vi "SmartSyntax to FormatString.vi"(0 "functionbase in":refnum<class "functionbase.lvclass">, 5 "String":string, 11 "error in (no error)":errorcluster) -> (4 "functionbase out":refnum<class "functionbase.lvclass">, 6 "Scan Syntax Format":T1, 15 "error out":errorcluster)   [LabVIEW 2019, in "LSL.lvlib" / "functionbase.lvclass"]
uses:
  functionbase.lvclass
  common/function utils/Scan Syntax Format.ctl
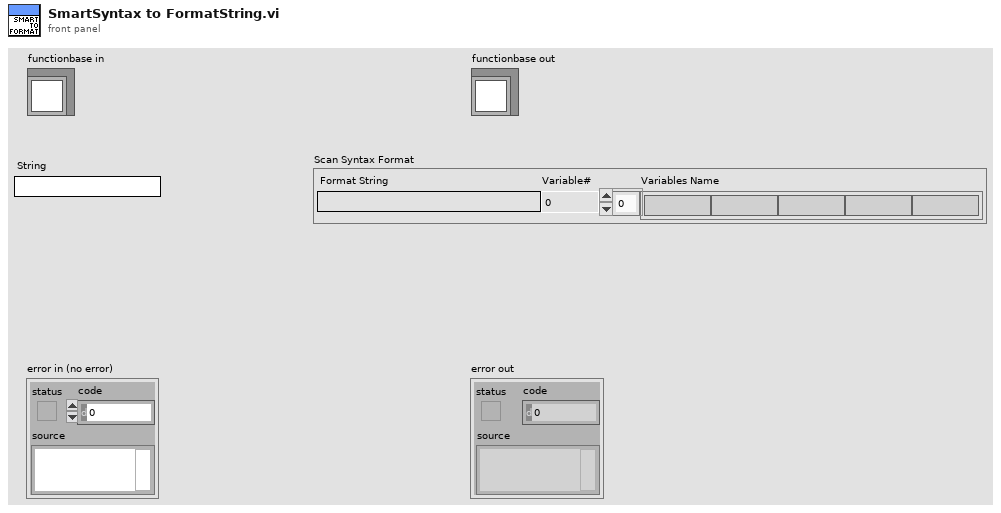
[diagram p1: front panel]
types:
  T1 = typedef "Scan Syntax Format.ctl" = cluster{"Format String":string, "Variable#":i32, "Variables Name":string[]}
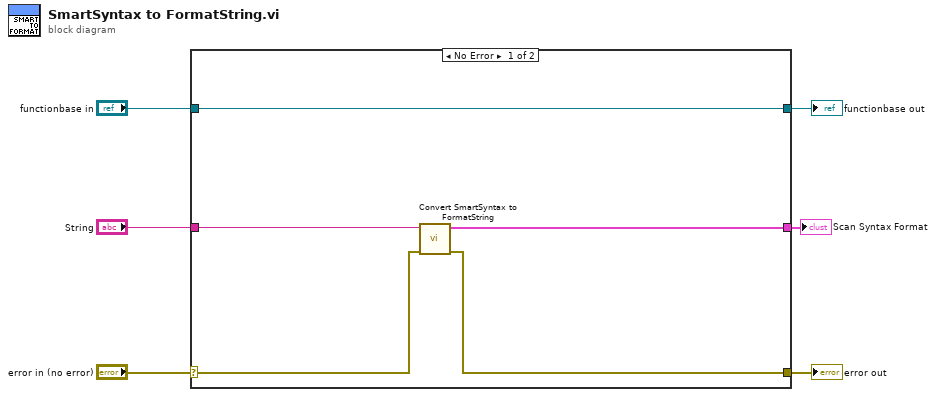
[diagram p0: block diagram]
diagram:
  n1 = case shown="No Error" "error in (no error)" {
    selector: "error in (no error)" -> [w9 w13]
    tunnel: [w8 w13] -> w5
    tunnel: [w11 w12] -> w3
    tunnel: "functionbase in" -> [w11 w12]
    tunnel: "String" -> [w10 _]
    tunnel: [w7 _] -> w1
    frame No Error {
      n2 = call "Convert SmartSyntax to FormatString.vi"("error in (no error)"=w9, "Smart Syntax"=w10) -> ("error out"=w8:errorcluster, "Scan Syntax Format"=w7:T1)  [unwired: 8 in]
    }
    frame Error {
    }
  }
  "error out" <- w5
  "functionbase out" <- w3
  "Scan Syntax Format" <- w1
